vi "Begin.vi"(8 "error in":errorcluster) -> (0 "error out":errorcluster)   [LabVIEW 2019]
doc: "Called before other user functions, this VI can be used to open I/O refnums, load in file data, and do general program initialization. Notice that the <B>error out</B> terminal is simply used for data flow. Wiring it to other structures or subVIs ensures that this VI runs first."
uses:
  <vilib>/Rock Robotics/WPI/DriverStation/WPI_DriverStationRobotMode2.ctl
  <vilib>/Rock Robotics/WPI/Joystick/WPI_JoystickDeviceEnum.ctl
  <vilib>/Rock Robotics/SystemInterfaces/DIO/FPGA_DIOPWMChannel.ctl
  <vilib>/Rock Robotics/WPI/SafetyOutput/WPI_SafetyOutputConfigMenu.ctl
  <vilib>/Rock Robotics/WPI/Solenoid/WPI_SolenoidChannel.ctl
  <vilib>/Rock Robotics/SystemInterfaces/i2clib/i2c_bus.ctl
  <vilib>/Rock Robotics/WPI/Solenoid/WPI_SolenoidValue.ctl
  Robot Global Data.vi
  <vilib>/Rock Robotics/WPI/RobotDrive/WPI_RobotDriveOpen2MotorWithExistingMotors.vi
  <vilib>/Rock Robotics/WPI/MotorControl/WPI_MotorControlOpen SPARK.vi
  <vilib>/Rock Robotics/WPI/Solenoid/WPI_SolenoidOpenDouble.vi
  <vilib>/Rock Robotics/WPI/Solenoid/WPI_SolenoidSetEnum.vi
  <vilib>/Rock Robotics/Network Tables/NT Write Number.vi
  <vilib>/Rock Robotics/Network Tables/NT Write Boolean Array.vi
  <vilib>/Rock Robotics/Network Tables/NT Write Numeric Array.vi
panel:
  in  "Blue Calibration":cluster{"R":dbl, "G":dbl, "B":dbl}={"R"=0.143, "G"=0.427, "B"=0.429}
  in  "Green Calibration":cluster{"R":dbl, "G":dbl, "B":dbl}={"R"=0.197, "G"=0.561, "B"=0.24}
  in  "Red Calibration":cluster{"R":dbl, "G":dbl, "B":dbl}={"R"=0.561, "G"=0.323, "B"=0.114}
  in  "Yellow Calibration":cluster{"R":dbl, "G":dbl, "B":dbl}={"R"=0.361, "G"=0.524, "B"=0.113}
  in  "Calibration Time (sec)":u32=4
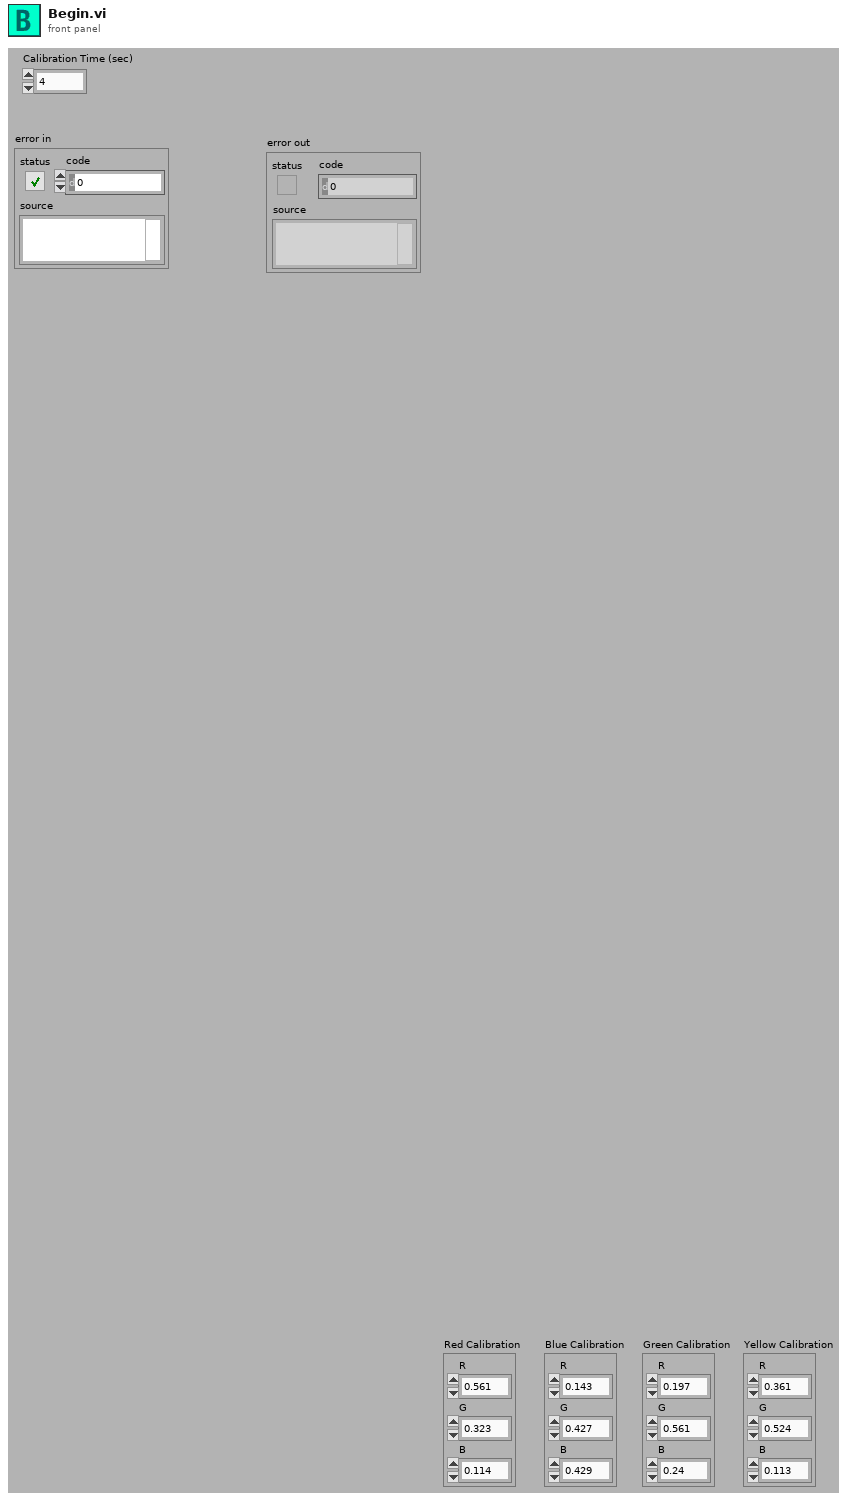
[diagram p1: front panel]
types:
  T1 = typedef "WPI_SolenoidChannel.ctl" = enum8{"Solenoid 0", "Solenoid 1", "Solenoid 2", "Solenoid 3", "Solenoid 4", "Solenoid 5", "Solenoid 6", "Solenoid 7", "Invalid"}
  T2 = typedef "WPI_SolenoidValue.ctl" = enum16{"Off", "On", "Forward", "Reverse"}
  T3 = typedef "WPI_SafetyOutputConfigMenu.ctl" = enum16{"Enable", "Disable"}
  T4 = typedef "i2c_bus.ctl" = enum16{"I2C On-Board", "I2C MXP", "Invalid"}
  T5 = typedef "FPGA_DIOPWMChannel.ctl" = enum8{"PWM 0", "PWM 1", "PWM 2", "PWM 3", "PWM 4", "PWM 5", "PWM 6", "PWM 7", "PWM 8", "PWM 9", "PWM MXP 0", "PWM MXP 1", "PWM MXP 2", "PWM MXP 3", "PWM MXP 4", "PWM MXP 5", "PWM MXP 6", "PWM MXP 7", "PWM MXP 8", "PWM MXP 9", "Invalid"}
  T6 = typedef "WPI_JoystickDeviceEnum.ctl" = enum16{"USB 0", "USB 1", "USB 2", "USB 3", "USB 4", "USB 5"}
  T7 = typedef "WPI_DriverStationRobotMode2.ctl" = enum16{"Autonomous Disabled", "Autonomous Enabled", "Teleop Disabled", "Teleop Enabled", "Disconnected", "Finish", "Test Disabled", "Test Enabled", "Emergency Stopped"}
  T8 = typedef "WPI_JoystickDevRef.ctl" = cluster{"Device":T6}
  T9 = typedef "WPI_MotorControlDeviceRef.ctl" = cluster{"DeviceStatus":errorcluster, "Type":T10, "PWM":cluster{"PWM Channel":T5, "DeadBand":T11}, "CAN":cluster{"Device Number":u8, "SetOutput VI Ref":variant, "GetOutput VI Ref":variant, "Enable VI Ref":variant, "Disable VI Ref":variant, "Data":variant}, "Invert":bool, "DIO PWM":cluster{"PWM \"Enable\" Channel":T5, "DIOChannel":T12, "PWM Rate":dbl}}
  T10 = typedef "WPI_MotorControlType.ctl" = enum16{"PWM", "CAN", "DIO PWM"}
  T11 = typedef "WPI_PWMDeadband.ctl" = cluster{"Name":string, "maxPositivePwm":i32, "minPositivePwm":i32, "centerPwm":i32, "maxNegativePwm":i32, "minNegativePwm":i32, "angularRange":u16}
  T12 = typedef "FPGA_DIOChannel.ctl" = enum8{"DIO 0", "DIO 1", "DIO 2", "DIO 3", "DIO 4", "DIO 5", "DIO 6", "DIO 7", "DIO 8", "DIO 9", "DIO MXP 0", "DIO MXP 1", "DIO MXP 2", "DIO MXP 3", "DIO MXP 4", "DIO MXP 5", "DIO MXP 6", "DIO MXP 7", "DIO MXP 8", "DIO MXP 9", "DIO MXP 10", "DIO MXP 11", "DIO MXP 12", "DIO MXP 13", "DIO MXP 14", "DIO MXP 15", "SPI Port CS1", "SPI Port CS2", "SPI Port CS3", "SPI Port MISO", "SPI Port MOSI", "Invalid"}
  T13 = typedef "WPI_RobotDriveDevRef.ctl" = cluster{"DevStatus":errorcluster, "Motors[]":T9[], "Square Inputs":bool, "Max Output":dbl}
  T14 = typedef "Color Sensor V3 DevRef.ctl" = cluster{"I2CDevRef":T15}
  T15 = typedef "WPI_I2CDevRef.ctl" = cluster{"DevStatus":errorcluster, "Device Address":u8, "Handle":i32, "I2C Bus":T4}
  T16 = typedef "WPI_SolenoidDevRef.ctl" = cluster{"DevStatus":errorcluster, "Pneumatics Control Module":u8, "Forward Solenoid Channel":T1, "Reverse Solenoid Channel":T1}
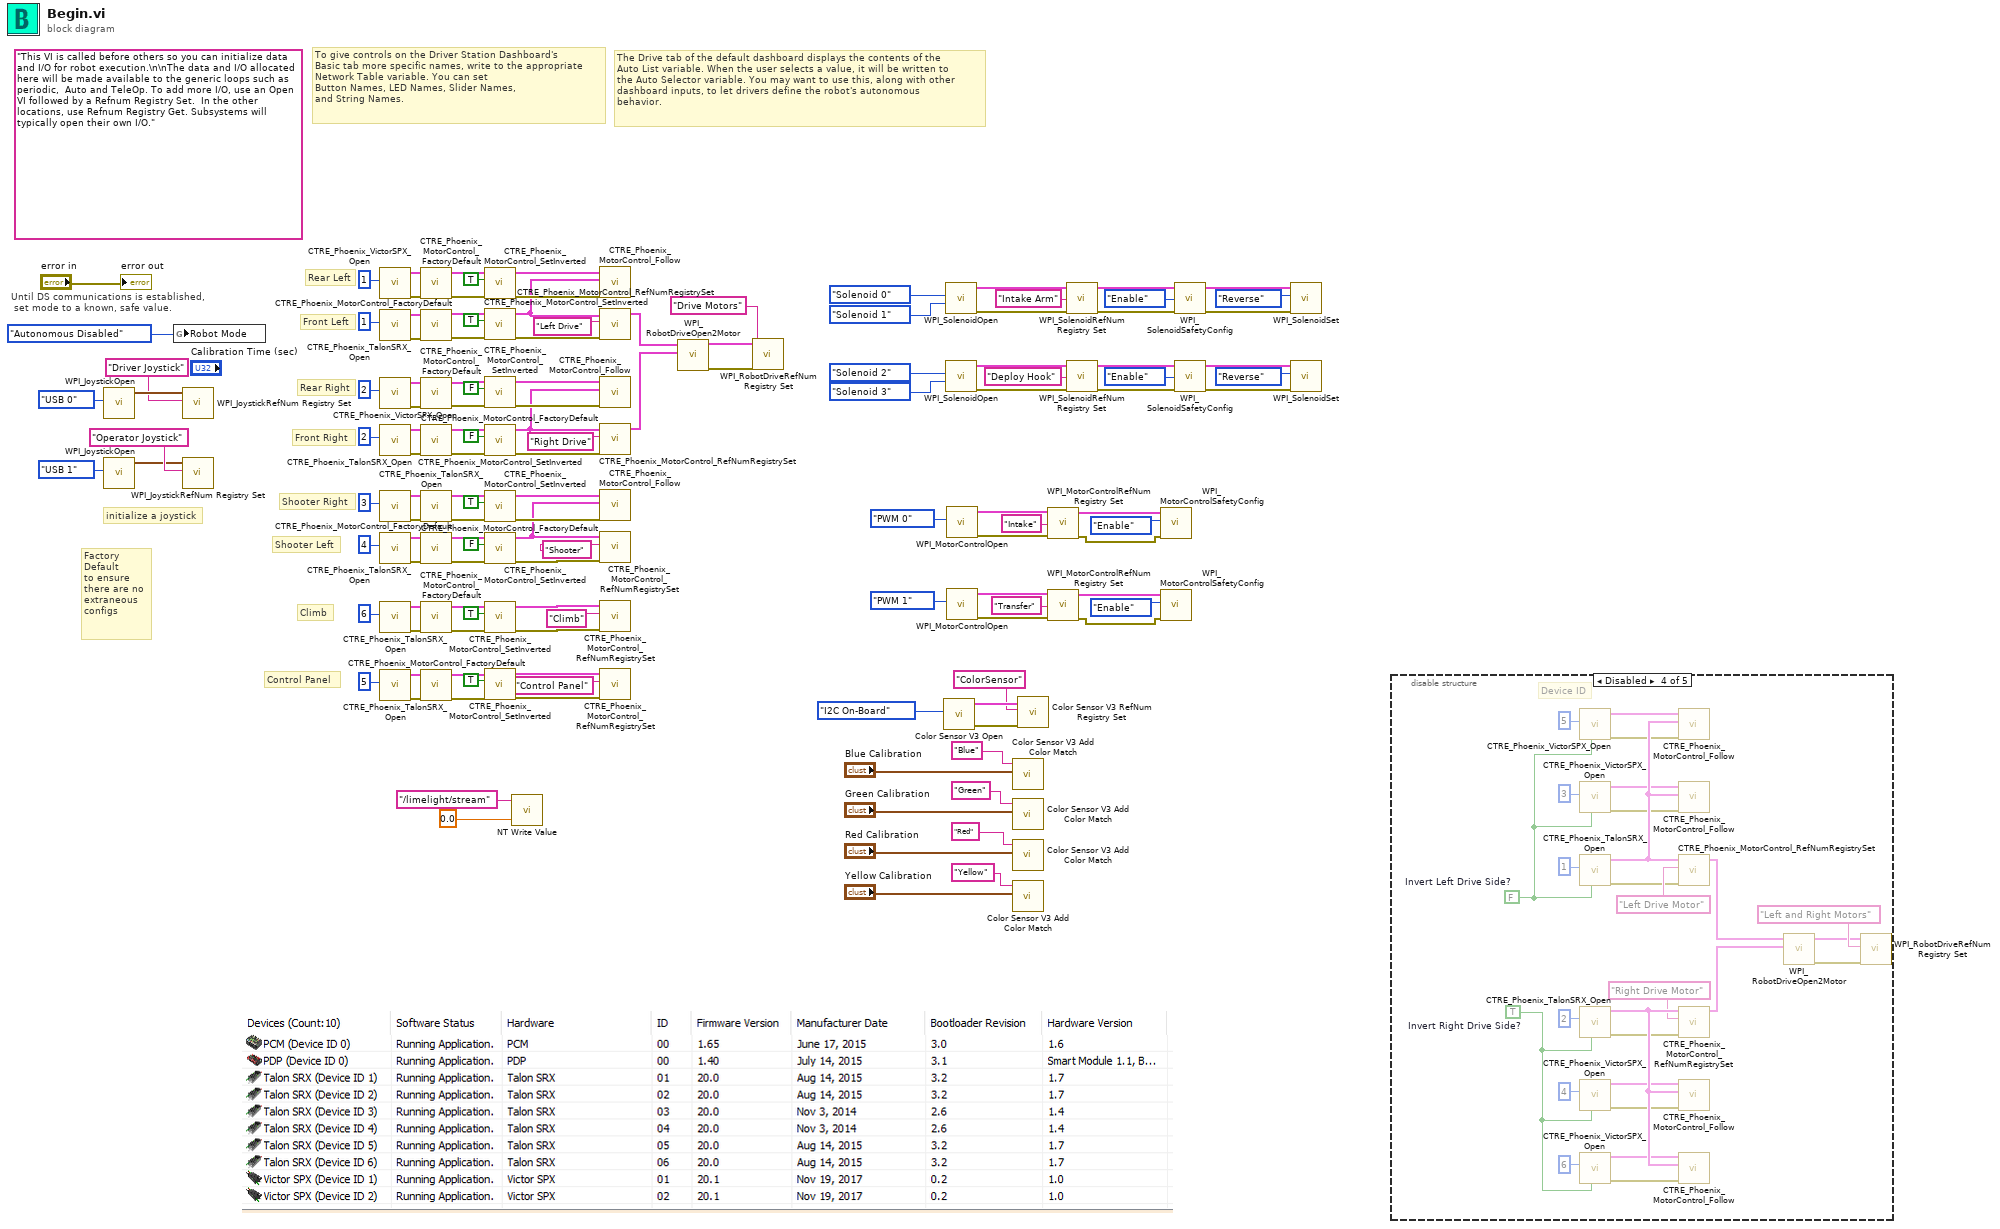
[diagram p0: block diagram]
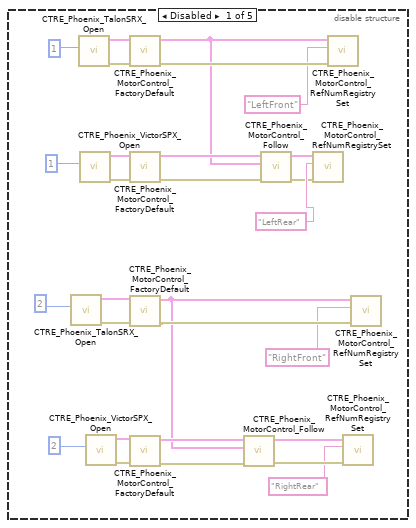
[diagram p2: hidden frame]
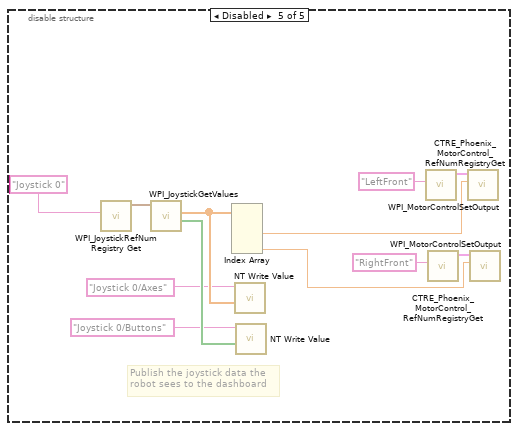
[diagram p5: hidden frame]
diagram:
  (unwired) "This VI is called before others so you can initialize data and I/O for robot execution.\n\nThe data and I/O allocated here will be made available to the generic loops such as periodic,  Auto and TeleOp. To add more I/O, use an Open VI followed by a Refnum Registry Set.  In the other locations, use Refnum Registry Get. Subsystems will typically open their own I/O."
  # "Climb"
  # "Control Panel"
  # "The Drive tab of the default dashboard displays the contents of the\nAuto List variable. When the user selects a value, it will be written to\nthe Auto Selector variable. You may want to use this, along with other\ndashboard inputs, to let drivers define the robot's autonomous\nbehavior."
  # "To give controls on the Driver Station Dashboard's\nBasic tab more specific names, write to the appropriate\nNetwork Table variable. You can set\nButton Names, LED Names, Slider Names,\nand String Names."
  # "Shooter Left"
  # "Shooter Right"
  # "Factory \nDefault \nto ensure \nthere are no \nextraneous \nconfigs"
  # "Front Right"
  # "Front Left"
  # "Rear Right"
  # "Rear Left"
  # "initialize a joystick"
  # "Until DS communications is established,\n set mode to a known, safe value."
  n1 = call <vilib>:"WPI_JoystickOpen.vi"("JoystickDevice"=WPI_JoystickDeviceEnum."USB 0") -> ("JoystickDevRef"=w115:T8)  [unwired: 10 in]
  n2 = call <vilib>:"WPI_JoystickOpen.vi"("JoystickDevice"=WPI_JoystickDeviceEnum."USB 1") -> ("JoystickDevRef"=w130:T8)  [unwired: 10 in]
  n3 = global write "Robot Global Data.vi" "Robot Mode"(WPI_DriverStationRobotMode2."Autonomous Disabled" ("Robot Mode")) -> ()
  n4 = call <vilib>:"WPI_JoystickRefNum Registry Set.vi"("refnum name"="Driver Joystick", "JoystickDevRef"=w115) -> ()  [unwired: 8 in, 2 out]
  n5 = call <vilib>:"WPI_JoystickRefNum Registry Set.vi"("refnum name"="Operator Joystick", "JoystickDevRef"=w130) -> ()  [unwired: 8 in, 2 out]
  n6 = call <vilib>:"CTRE_Phoenix_VictorSPX_Open.vi"("Device Number"=u8 1) -> ("error out"=w113:errorcluster, "CAN Talon SRX Ref"=w112:T9)  [unwired: 9 in]
  n7 = call <vilib>:"CTRE_Phoenix_TalonSRX_Open.vi"("Device Number"=u8 1) -> ("error out"=w110:errorcluster, "CAN Talon SRX Ref"=w111:T9)  [unwired: 9 in]
  n8 = call <vilib>:"CTRE_Phoenix_VictorSPX_Open.vi"("Device Number"=u8 2) -> ("error out"=w109:errorcluster, "CAN Talon SRX Ref"=w108:T9)  [unwired: 9 in]
  n9 = call <vilib>:"CTRE_Phoenix_TalonSRX_Open.vi"("Device Number"=u8 2) -> ("error out"=w107:errorcluster, "CAN Talon SRX Ref"=w106:T9)  [unwired: 9 in]
  n10 = call <vilib>:"CTRE_Phoenix_TalonSRX_Open.vi"("Device Number"=u8 3) -> ("error out"=w68:errorcluster, "CAN Talon SRX Ref"=w67:T9)  [unwired: 9 in]
  n11 = call <vilib>:"CTRE_Phoenix_TalonSRX_Open.vi"("Device Number"=u8 4) -> ("error out"=w66:errorcluster, "CAN Talon SRX Ref"=w65:T9)  [unwired: 9 in]
  n12 = call <vilib>:"CTRE_Phoenix_TalonSRX_Open.vi"("Device Number"=u8 6) -> ("error out"=w7:errorcluster, "CAN Talon SRX Ref"=w6:T9)  [unwired: 9 in]
  n13 = call <vilib>:"CTRE_Phoenix_TalonSRX_Open.vi"("Device Number"=u8 5) -> ("error out"=w41:errorcluster, "CAN Talon SRX Ref"=w40:T9)  [unwired: 9 in]
  n14 = call <vilib>:"CTRE_Phoenix_MotorControl_FactoryDefault.vi"("error in"=w113, "PhoenixMotorControlDevRef"=w112) -> ("error out"=w104:errorcluster, "PhoenixMotorControlDevRef"=w103:T9)  [unwired: 8 in]
  n15 = call <vilib>:"CTRE_Phoenix_MotorControl_FactoryDefault.vi"("error in"=w110, "PhoenixMotorControlDevRef"=w111) -> ("error out"=w98:errorcluster, "PhoenixMotorControlDevRef"=w99:T9)  [unwired: 8 in]
  n16 = call <vilib>:"CTRE_Phoenix_MotorControl_FactoryDefault.vi"("error in"=w109, "PhoenixMotorControlDevRef"=w108) -> ("error out"=w94:errorcluster, "PhoenixMotorControlDevRef"=w93:T9)  [unwired: 8 in]
  n17 = call <vilib>:"CTRE_Phoenix_MotorControl_FactoryDefault.vi"("error in"=w107, "PhoenixMotorControlDevRef"=w106) -> ("error out"=w89:errorcluster, "PhoenixMotorControlDevRef"=w88:T9)  [unwired: 8 in]
  n18 = call <vilib>:"CTRE_Phoenix_MotorControl_FactoryDefault.vi"("error in"=w68, "PhoenixMotorControlDevRef"=w67) -> ("error out"=w62:errorcluster, "PhoenixMotorControlDevRef"=w63:T9)  [unwired: 8 in]
  n19 = call <vilib>:"CTRE_Phoenix_MotorControl_FactoryDefault.vi"("error in"=w66, "PhoenixMotorControlDevRef"=w65) -> ("error out"=w57:errorcluster, "PhoenixMotorControlDevRef"=w58:T9)  [unwired: 8 in]
  n20 = call <vilib>:"CTRE_Phoenix_MotorControl_FactoryDefault.vi"("error in"=w7, "PhoenixMotorControlDevRef"=w6) -> ("error out"=w3:errorcluster, "PhoenixMotorControlDevRef"=w4:T9)  [unwired: 8 in]
  n21 = call <vilib>:"CTRE_Phoenix_MotorControl_FactoryDefault.vi"("error in"=w41, "PhoenixMotorControlDevRef"=w40) -> ("error out"=w37:errorcluster, "PhoenixMotorControlDevRef"=w38:T9)  [unwired: 8 in]
  n22 = call <vilib>:"CTRE_Phoenix_MotorControl_SetInverted.vi"("error in (no error)"=w104, "Invert?"=TRUE, "PhoenixMotorControlDevRef"=w103) -> ("error out"=w101:errorcluster, "PhoenixMotorControlDevRef"=w102:T9)  [unwired: 7 in]
  n23 = call <vilib>:"CTRE_Phoenix_MotorControl_SetInverted.vi"("error in (no error)"=w98, "Invert?"=TRUE, "PhoenixMotorControlDevRef"=w99) -> ("error out"=w97:errorcluster, "PhoenixMotorControlDevRef"=w96:T9)  [unwired: 7 in]
  n24 = call <vilib>:"CTRE_Phoenix_MotorControl_SetInverted.vi"("error in (no error)"=w94, "Invert?"=FALSE, "PhoenixMotorControlDevRef"=w93) -> ("error out"=w91:errorcluster, "PhoenixMotorControlDevRef"=w92:T9)  [unwired: 7 in]
  n25 = call <vilib>:"CTRE_Phoenix_MotorControl_SetInverted.vi"("error in (no error)"=w89, "Invert?"=FALSE, "PhoenixMotorControlDevRef"=w88) -> ("error out"=w86:errorcluster, "PhoenixMotorControlDevRef"=w87:T9)  [unwired: 7 in]
  n26 = call <vilib>:"CTRE_Phoenix_MotorControl_SetInverted.vi"("error in (no error)"=w62, "Invert?"=TRUE, "PhoenixMotorControlDevRef"=w63) -> ("error out"=w61:errorcluster, "PhoenixMotorControlDevRef"=w60:T9)  [unwired: 7 in]
  n27 = call <vilib>:"CTRE_Phoenix_MotorControl_SetInverted.vi"("error in (no error)"=w57, "Invert?"=FALSE, "PhoenixMotorControlDevRef"=w58) -> ("error out"=w56:errorcluster, "PhoenixMotorControlDevRef"=w55:T9)  [unwired: 7 in]
  n28 = call <vilib>:"CTRE_Phoenix_MotorControl_SetInverted.vi"("error in (no error)"=w3, "Invert?"=TRUE, "PhoenixMotorControlDevRef"=w4) -> ("error out"=w2:errorcluster, "PhoenixMotorControlDevRef"=w1:T9)  [unwired: 7 in]
  n29 = call <vilib>:"CTRE_Phoenix_MotorControl_SetInverted.vi"("error in (no error)"=w37, "Invert?"=TRUE, "PhoenixMotorControlDevRef"=w38) -> ("error out"=w36:errorcluster, "PhoenixMotorControlDevRef"=w35:T9)  [unwired: 7 in]
  n30 = call-poly <vilib>:"NT Write Value.vi"("Numeric"=0.0, "Name"="/limelight/stream") -> ()  [unwired: 9 in, 1 out]
  n31 = call <vilib>:"CTRE_Phoenix_MotorControl_Follow.vi"("error in (no error)"=w101, "Master Controller to Follow"=w96, "PhoenixMotorControlDevRef"=w102) -> ()  [unwired: 7 in, 2 out]
  n32 = call <vilib>:"CTRE_Phoenix_MotorControl_RefNumRegistrySet.vi"("error in (no error)"=w97, "refnum name"="Left Drive", "PhoenixMotorControlDevRef"=w96) -> ("PhoenixMotorControlDevRef"=w123:T9)  [unwired: 7 in, 1 out]
  n33 = call <vilib>:"CTRE_Phoenix_MotorControl_Follow.vi"("error in (no error)"=w91, "Master Controller to Follow"=w87, "PhoenixMotorControlDevRef"=w92) -> ()  [unwired: 7 in, 2 out]
  n34 = call <vilib>:"CTRE_Phoenix_MotorControl_RefNumRegistrySet.vi"("error in (no error)"=w86, "refnum name"="Right Drive", "PhoenixMotorControlDevRef"=w87) -> ("PhoenixMotorControlDevRef"=w122:T9)  [unwired: 7 in, 1 out]
  n35 = call <vilib>:"CTRE_Phoenix_MotorControl_Follow.vi"("error in (no error)"=w61, "Master Controller to Follow"=w55, "PhoenixMotorControlDevRef"=w60) -> ()  [unwired: 7 in, 2 out]
  n36 = call <vilib>:"CTRE_Phoenix_MotorControl_RefNumRegistrySet.vi"("error in (no error)"=w56, "refnum name"="Shooter", "PhoenixMotorControlDevRef"=w55) -> ()  [unwired: 7 in, 2 out]
  n37 = call <vilib>:"CTRE_Phoenix_MotorControl_RefNumRegistrySet.vi"("error in (no error)"=w2, "refnum name"="Climb", "PhoenixMotorControlDevRef"=w1) -> ()  [unwired: 7 in, 2 out]
  n38 = call <vilib>:"CTRE_Phoenix_MotorControl_RefNumRegistrySet.vi"("error in (no error)"=w36, "refnum name"="Control Panel", "PhoenixMotorControlDevRef"=w35) -> ()  [unwired: 7 in, 2 out]
  n39 = call-poly <vilib>:"WPI_RobotDriveOpen2Motor.vi"("Right Motor Dev Ref"=w122, "Left Motor Dev Ref"=w123) -> ("error out"=w118:errorcluster, "RobotDriveDevRef"=w119:T13)  [unwired: 8 in]
  n40 = call <vilib>:"WPI_RobotDriveRefNum Registry Set.vi"("error in (no error)"=w118, "refnum name"="Drive Motors", "RobotDriveDevRef"=w119) -> ()  [unwired: 7 in, 2 out]
  n41 = call <vilib>:"Color Sensor V3 Open.vi"("I2C Bus"=i2c_bus."I2C On-Board") -> ("error out"=w32:errorcluster, "ColorSensorDevRef"=w33:T14)  [unwired: 9 in]
  n42 = call-poly <vilib>:"WPI_SolenoidOpen.vi"("Reverse Solenoid Channel"=WPI_SolenoidChannel."Solenoid 1" ("Solenoid Channel"), "Forward Solenoid Channel"=WPI_SolenoidChannel."Solenoid 0" ("Solenoid Channel")) -> ("error out"=w51:errorcluster, "SolenoidDevRef"=w54:T16)  [unwired: 8 in]
  n43 = call-poly <vilib>:"WPI_SolenoidOpen.vi"("Reverse Solenoid Channel"=WPI_SolenoidChannel."Solenoid 3" ("Solenoid Channel"), "Forward Solenoid Channel"=WPI_SolenoidChannel."Solenoid 2" ("Solenoid Channel")) -> ("error out"=w14:errorcluster, "SolenoidDevRef"=w11:T16)  [unwired: 8 in]
  n44 = call-poly <vilib>:"WPI_MotorControlOpen.vi"("PWM Channel"=FPGA_DIOPWMChannel."PWM 0") -> ("error out"=w80:errorcluster, "MotorControlDeviceRef"=w84:T9)  [unwired: 9 in]
  n45 = call-poly <vilib>:"WPI_MotorControlOpen.vi"("PWM Channel"=FPGA_DIOPWMChannel."PWM 1") -> ("error out"=w77:errorcluster, "MotorControlDeviceRef"=w73:T9)  [unwired: 9 in]
  n46 = call <vilib>:"Color Sensor V3 Add Color Match.vi"("Color"="Blue Calibration", "Name"="Blue") -> ()  [unwired: 10 in]
  n47 = call <vilib>:"Color Sensor V3 Add Color Match.vi"("Color"="Green Calibration", "Name"="Green") -> ()  [unwired: 10 in]
  n48 = call <vilib>:"Color Sensor V3 Add Color Match.vi"("Color"="Red Calibration", "Name"="Red") -> ()  [unwired: 10 in]
  n49 = call <vilib>:"Color Sensor V3 Add Color Match.vi"("Color"="Yellow Calibration", "Name"="Yellow") -> ()  [unwired: 10 in]
  n50 = call <vilib>:"Color Sensor V3 RefNum Registry Set.vi"("error in (no error)"=w32, "refnum name"="ColorSensor", "ColorSensorDevRef"=w33) -> ()  [unwired: 7 in, 2 out]
  n51 = call <vilib>:"WPI_MotorControlRefNum Registry Set.vi"("error in (no error)"=w80, "refnum name"="Intake", "MotorControlDevRef"=w84) -> ("error out"=w79:errorcluster, "MotorControlDevRef"=w83:T9)  [unwired: 7 in]
  n52 = call <vilib>:"WPI_MotorControlRefNum Registry Set.vi"("error in (no error)"=w77, "refnum name"="Transfer", "MotorControlDevRef"=w73) -> ("error out"=w78:errorcluster, "MotorControlDevRef"=w74:T9)  [unwired: 7 in]
  n53 = call <vilib>:"WPI_SolenoidRefNum Registry Set.vi"("error in (no error)"=w51, "refnum name"="Intake Arm", "SolenoidDevRef"=w54) -> ("error out"=w50:errorcluster, "SolenoidDevRef"=w53:T16)  [unwired: 7 in]
  n54 = call <vilib>:"WPI_SolenoidRefNum Registry Set.vi"("error in (no error)"=w14, "refnum name"="Deploy Hook", "SolenoidDevRef"=w11) -> ("error out"=w15:errorcluster, "SolenoidDevRef"=w12:T16)  [unwired: 7 in]
  n55 = call <vilib>:"WPI_MotorControlSafetyConfig.vi"("error in (no error)"=w79, "mode"=WPI_SafetyOutputConfigMenu."Enable", "MotorControlDevRef"=w83) -> ()  [unwired: 7 in, 2 out]
  n56 = call <vilib>:"WPI_MotorControlSafetyConfig.vi"("error in (no error)"=w78, "mode"=WPI_SafetyOutputConfigMenu."Enable", "MotorControlDevRef"=w74) -> ()  [unwired: 7 in, 2 out]
  n57 = call <vilib>:"WPI_SolenoidSafetyConfig.vi"("error in (no error)"=w50, "mode"=WPI_SafetyOutputConfigMenu."Enable", "SolenoidDevRef"=w53) -> ("error out"=w49:errorcluster, "SolenoidDevRef"=w52:T16)  [unwired: 7 in]
  n58 = call <vilib>:"WPI_SolenoidSafetyConfig.vi"("error in (no error)"=w15, "mode"=WPI_SafetyOutputConfigMenu."Enable", "SolenoidDevRef"=w12) -> ("error out"=w16:errorcluster, "SolenoidDevRef"=w13:T16)  [unwired: 7 in]
  n59 = call-poly <vilib>:"WPI_SolenoidSet.vi"("error in (no error)"=w49, "Value"=WPI_SolenoidValue."Reverse", "SolenoidDevRef"=w52) -> ()  [unwired: 7 in, 2 out]
  n60 = call-poly <vilib>:"WPI_SolenoidSet.vi"("error in (no error)"=w16, "Value"=WPI_SolenoidValue."Reverse", "SolenoidDevRef"=w13) -> ()  [unwired: 7 in, 2 out]
  n61 = disable-structure shown="Disabled" {
    frame Disabled {
      n62 = call <vilib>:"CTRE_Phoenix_TalonSRX_Open.vi"("Device Number"=u8 2) -> ("error out"=w157:errorcluster, "CAN Talon SRX Ref"=w147:T9)  [unwired: 9 in]
      n63 = call <vilib>:"CTRE_Phoenix_TalonSRX_Open.vi"("Device Number"=u8 1) -> ("error out"=w155:errorcluster, "CAN Talon SRX Ref"=w145:T9)  [unwired: 9 in]
      n64 = call <vilib>:"CTRE_Phoenix_VictorSPX_Open.vi"("Device Number"=u8 1) -> ("error out"=w153:errorcluster, "CAN Talon SRX Ref"=w151:T9)  [unwired: 9 in]
      n65 = call <vilib>:"CTRE_Phoenix_VictorSPX_Open.vi"("Device Number"=u8 2) -> ("error out"=w159:errorcluster, "CAN Talon SRX Ref"=w149:T9)  [unwired: 9 in]
      n66 = call <vilib>:"CTRE_Phoenix_MotorControl_FactoryDefault.vi"("error in"=w155, "PhoenixMotorControlDevRef"=w145) -> ("error out"=w156:errorcluster, "PhoenixMotorControlDevRef"=w146:T9)  [unwired: 8 in]
      n67 = call <vilib>:"CTRE_Phoenix_MotorControl_FactoryDefault.vi"("error in"=w153, "PhoenixMotorControlDevRef"=w151) -> ("error out"=w154:errorcluster, "PhoenixMotorControlDevRef"=w152:T9)  [unwired: 8 in]
      n68 = call <vilib>:"CTRE_Phoenix_MotorControl_FactoryDefault.vi"("error in"=w157, "PhoenixMotorControlDevRef"=w147) -> ("error out"=w158:errorcluster, "PhoenixMotorControlDevRef"=w148:T9)  [unwired: 8 in]
      n69 = call <vilib>:"CTRE_Phoenix_MotorControl_FactoryDefault.vi"("error in"=w159, "PhoenixMotorControlDevRef"=w149) -> ("error out"=w160:errorcluster, "PhoenixMotorControlDevRef"=w150:T9)  [unwired: 8 in]
      n70 = call <vilib>:"CTRE_Phoenix_MotorControl_Follow.vi"("error in (no error)"=w160, "Master Controller to Follow"=w148, "PhoenixMotorControlDevRef"=w150) -> ("error out"=w143:errorcluster, "PhoenixMotorControlDevRef"=w144:T9)  [unwired: 7 in]
      n71 = call <vilib>:"CTRE_Phoenix_MotorControl_Follow.vi"("error in (no error)"=w154, "Master Controller to Follow"=w146, "PhoenixMotorControlDevRef"=w152) -> ("error out"=w135:errorcluster, "PhoenixMotorControlDevRef"=w136:T9)  [unwired: 7 in]
      n72 = call <vilib>:"CTRE_Phoenix_MotorControl_RefNumRegistrySet.vi"("error in (no error)"=w135, "refnum name"="LeftRear", "PhoenixMotorControlDevRef"=w136) -> ()  [unwired: 7 in, 2 out]
      n73 = call <vilib>:"CTRE_Phoenix_MotorControl_RefNumRegistrySet.vi"("error in (no error)"=w156, "refnum name"="LeftFront", "PhoenixMotorControlDevRef"=w146) -> ()  [unwired: 7 in, 2 out]
      n74 = call <vilib>:"CTRE_Phoenix_MotorControl_RefNumRegistrySet.vi"("error in (no error)"=w143, "refnum name"="RightRear", "PhoenixMotorControlDevRef"=w144) -> ()  [unwired: 7 in, 2 out]
      n75 = call <vilib>:"CTRE_Phoenix_MotorControl_RefNumRegistrySet.vi"("error in (no error)"=w158, "refnum name"="RightFront", "PhoenixMotorControlDevRef"=w148) -> ()  [unwired: 7 in, 2 out]
    }
    frame Enabled {
    }
    frame Disabled {
    }
    frame Disabled {
      w187 = FALSE  # Invert Left Drive Side?
      w186 = TRUE  # Invert Right Drive Side?
      # "Device ID"
      n76 = call <vilib>:"CTRE_Phoenix_VictorSPX_Open.vi"("Invert"=w187, "Device Number"=u8 5) -> ("error out"=w177:errorcluster, "CAN Talon SRX Ref"=w178:T9)  [unwired: 8 in]
      n77 = call <vilib>:"CTRE_Phoenix_VictorSPX_Open.vi"("Invert"=w187, "Device Number"=u8 3) -> ("error out"=w176:errorcluster, "CAN Talon SRX Ref"=w179:T9)  [unwired: 8 in]
      n78 = call <vilib>:"CTRE_Phoenix_TalonSRX_Open.vi"("Invert"=w187, "Device Number"=u8 1) -> ("error out"=w167:errorcluster, "CAN Talon SRX Ref"=w180:T9)  [unwired: 8 in]
      n79 = call <vilib>:"CTRE_Phoenix_TalonSRX_Open.vi"("Invert"=w186, "Device Number"=u8 2) -> ("error out"=w168:errorcluster, "CAN Talon SRX Ref"=w175:T9)  [unwired: 8 in]
      n80 = call <vilib>:"CTRE_Phoenix_VictorSPX_Open.vi"("Invert"=w186, "Device Number"=u8 4) -> ("error out"=w171:errorcluster, "CAN Talon SRX Ref"=w172:T9)  [unwired: 8 in]
      n81 = call <vilib>:"CTRE_Phoenix_VictorSPX_Open.vi"("Invert"=w186, "Device Number"=u8 6) -> ("error out"=w174:errorcluster, "CAN Talon SRX Ref"=w173:T9)  [unwired: 8 in]
      n82 = call <vilib>:"CTRE_Phoenix_MotorControl_Follow.vi"("error in (no error)"=w177, "Master Controller to Follow"=w180, "PhoenixMotorControlDevRef"=w178) -> ()  [unwired: 7 in, 2 out]
      n83 = call <vilib>:"CTRE_Phoenix_MotorControl_Follow.vi"("error in (no error)"=w176, "Master Controller to Follow"=w180, "PhoenixMotorControlDevRef"=w179) -> ()  [unwired: 7 in, 2 out]
      n84 = call <vilib>:"CTRE_Phoenix_MotorControl_RefNumRegistrySet.vi"("error in (no error)"=w167, "refnum name"="Left Drive Motor", "PhoenixMotorControlDevRef"=w180) -> ("PhoenixMotorControlDevRef"=w181:T9)  [unwired: 7 in, 1 out]
      n85 = call <vilib>:"CTRE_Phoenix_MotorControl_RefNumRegistrySet.vi"("error in (no error)"=w168, "refnum name"="Right Drive Motor", "PhoenixMotorControlDevRef"=w175) -> ("PhoenixMotorControlDevRef"=w182:T9)  [unwired: 7 in, 1 out]
      n86 = call <vilib>:"CTRE_Phoenix_MotorControl_Follow.vi"("error in (no error)"=w171, "Master Controller to Follow"=w175, "PhoenixMotorControlDevRef"=w172) -> ()  [unwired: 7 in, 2 out]
      n87 = call <vilib>:"CTRE_Phoenix_MotorControl_Follow.vi"("error in (no error)"=w174, "Master Controller to Follow"=w175, "PhoenixMotorControlDevRef"=w173) -> ()  [unwired: 7 in, 2 out]
      n88 = call-poly <vilib>:"WPI_RobotDriveOpen2Motor.vi"("Right Motor Dev Ref"=w182, "Left Motor Dev Ref"=w181) -> ("error out"=w183:errorcluster, "RobotDriveDevRef"=w184:T13)  [unwired: 8 in]
      n89 = call <vilib>:"WPI_RobotDriveRefNum Registry Set.vi"("error in (no error)"=w183, "refnum name"="Left and Right Motors", "RobotDriveDevRef"=w184) -> ()  [unwired: 7 in, 2 out]
    }
    frame Disabled {
      # "Publish the joystick data the\nrobot sees to the dashboard"
      n90 = call <vilib>:"WPI_JoystickRefNum Registry Get.vi"("refnum name"="Joystick 0") -> ("JoystickDevRef"=w189:T8)  [unwired: 1 in, 9 out]
      n91 = call <vilib>:"WPI_JoystickGetValues.vi"("JoystickDevRef"=w189) -> ("Buttons"=w193:bool[], "Axes"=w192:dbl[])  [unwired: 6 in, 3 out]
      n92 = Index Array(array=w192) -> (element #2=w196:dbl, element #4=w199:dbl)  [unwired: 4 in, 2 out]
      n93 = call-poly <vilib>:"NT Write Value.vi"("Numeric Array"=w192, "Name"="Joystick 0/Axes") -> ()  [unwired: 9 in, 1 out]
      n94 = call-poly <vilib>:"NT Write Value.vi"("Boolean Array"=w193, "Name"="Joystick 0/Buttons") -> ()  [unwired: 9 in, 1 out]
      n95 = call <vilib>:"CTRE_Phoenix_MotorControl_RefNumRegistryGet.vi"("refnum name"="LeftFront") -> ("PhoenixMotorControlDevRef"=w195:T9)  [unwired: 9 in, 1 out]
      n96 = call <vilib>:"CTRE_Phoenix_MotorControl_RefNumRegistryGet.vi"("refnum name"="RightFront") -> ("PhoenixMotorControlDevRef"=w198:T9)  [unwired: 9 in, 1 out]
      n97 = call <vilib>:"WPI_MotorControlSetOutput.vi"("Output"=w196, "MotorControlDevRef"=w195) -> ()  [unwired: 7 in, 3 out]
      n98 = call <vilib>:"WPI_MotorControlSetOutput.vi"("Output"=w199, "MotorControlDevRef"=w198) -> ()  [unwired: 7 in, 3 out]
    }
  }
  "error out" <- "error in"
